vi "LEDs.vi"(8 "error out":errorcluster) -> ()   [LabVIEW 2019]
uses:
  <vilib>/Rock Robotics/SystemInterfaces/DIO/FPGA_DIOPWMChannel.ctl
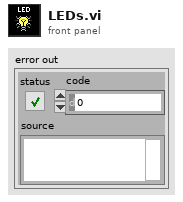
[diagram p1: front panel]
types:
  T1 = typedef "FPGA_DIOPWMChannel.ctl" = enum8{"PWM 0", "PWM 1", "PWM 2", "PWM 3", "PWM 4", "PWM 5", "PWM 6", "PWM 7", "PWM 8", "PWM 9", "PWM MXP 0", "PWM MXP 1", "PWM MXP 2", "PWM MXP 3", "PWM MXP 4", "PWM MXP 5", "PWM MXP 6", "PWM MXP 7", "PWM MXP 8", "PWM MXP 9", "Invalid"}
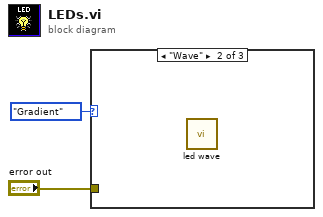
[diagram p0: block diagram]
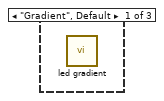
[diagram p2: hidden frame]
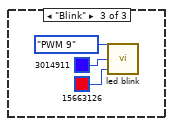
[diagram p3: hidden frame]
diagram:
  n1 = case shown="\"Wave\"" enum16{"Gradient", "Wave", "Blink"}."Gradient" ("LEDs") {
    tunnel: "error out" -> [_ _ _]
    frame "Gradient", Default {
      n2 = call "led gradient.vi"() -> ()  [unwired: 12 in]
    }
    frame "Wave" {
      n3 = call "led wave.vi"() -> ()  [unwired: 12 in]
    }
    frame "Blink" {
      n4 = call "led blink.vi"("Color Box 2"=u32 15663126, "Color Box"=u32 3014911, "PWM Channel"=FPGA_DIOPWMChannel."PWM 9") -> ()  [unwired: 5 in, 1 out]
    }
  }
